vi "Eurotherm_PID.vi"() -> ()   [LabVIEW 2013]
uses:
  <vilib>/Utility/file.llb/Write To Spreadsheet File (string).vi
  <vilib>/Utility/file.llb/Write To Spreadsheet File (DBL).vi
panel:
  in  "Thermocouple\nType":u8(ring)=1 items=["J.tc", "K.tc", "L.tc", "R.tc", "B.tc", "N.tc", "T.tc", "S.tc", "PL2.tc", "C.tc", "RTD", "Lin.mV", "Lin.V", "Lin.mA", "Sr.V", "Sr.mA", "mV.C", "V.C", "mA.C"]
  in  "Ramp-Down Rate(°C/ min)":dbl
  in  "Target Setpoint (°C)":sgl format="%#.1f"
  in  "RAMP":bool
  in  "Dwell Time (min)":dbl
  in  "Ramp-Up Rate (°C/ min)":dbl
  in  "SET":bool
  in  "DELAY":u32=300 caption="ms"
  in  "Save Button":bool
  in  "File Path":path
  in  "Sample":string
  in  "User":string
  out "Time":dbl caption="(s)"
  in  "Setpoint Value":sgl min=0 max=1300 format="%.3f"
  in  "SET":bool
  in  "P":sgl=1.0
  in  "I":u32=10000
  in  "D":u32=1000
  in  "Controller Mode":u8(ring) items=["Auto", "Manual"]
  in  "stop":bool
  out "Temperature":cluster{dbl[], sgl[]}(graph)
  out "Temperature":sgl caption="°C" format="%.3g"
  in  "Unit":u8=1
  in  "VISA resource name":refnum<visa-resource-name>="COM4"
  # "Configuration - Requires Restart"
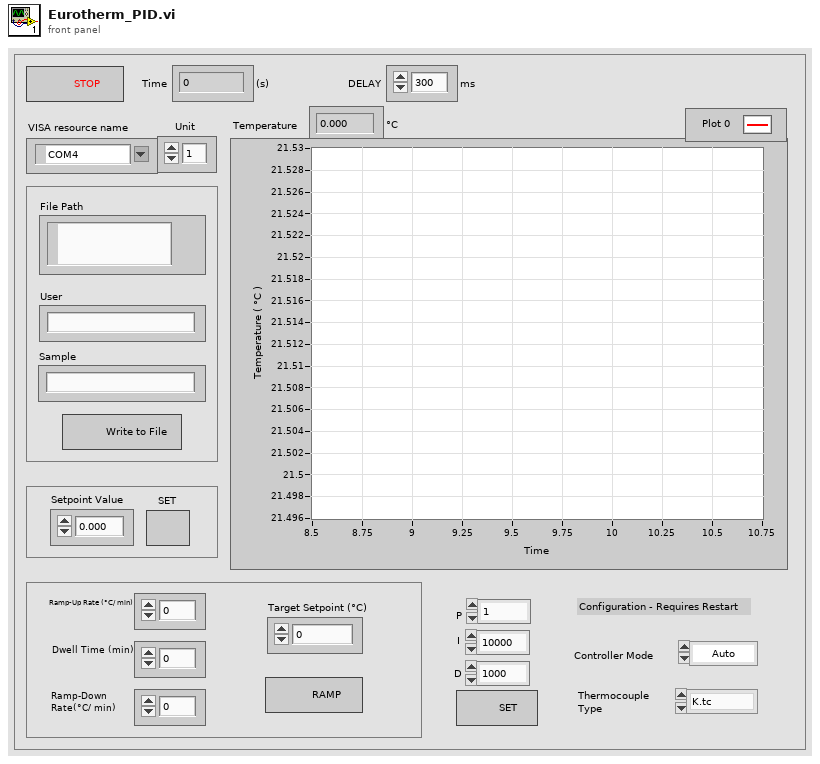
[diagram p1: front panel]
types:
  T1 = cluster{"Baud Rate (9600)":u32, "Parity (0: None)":u16, "Break Length (0)":u16}
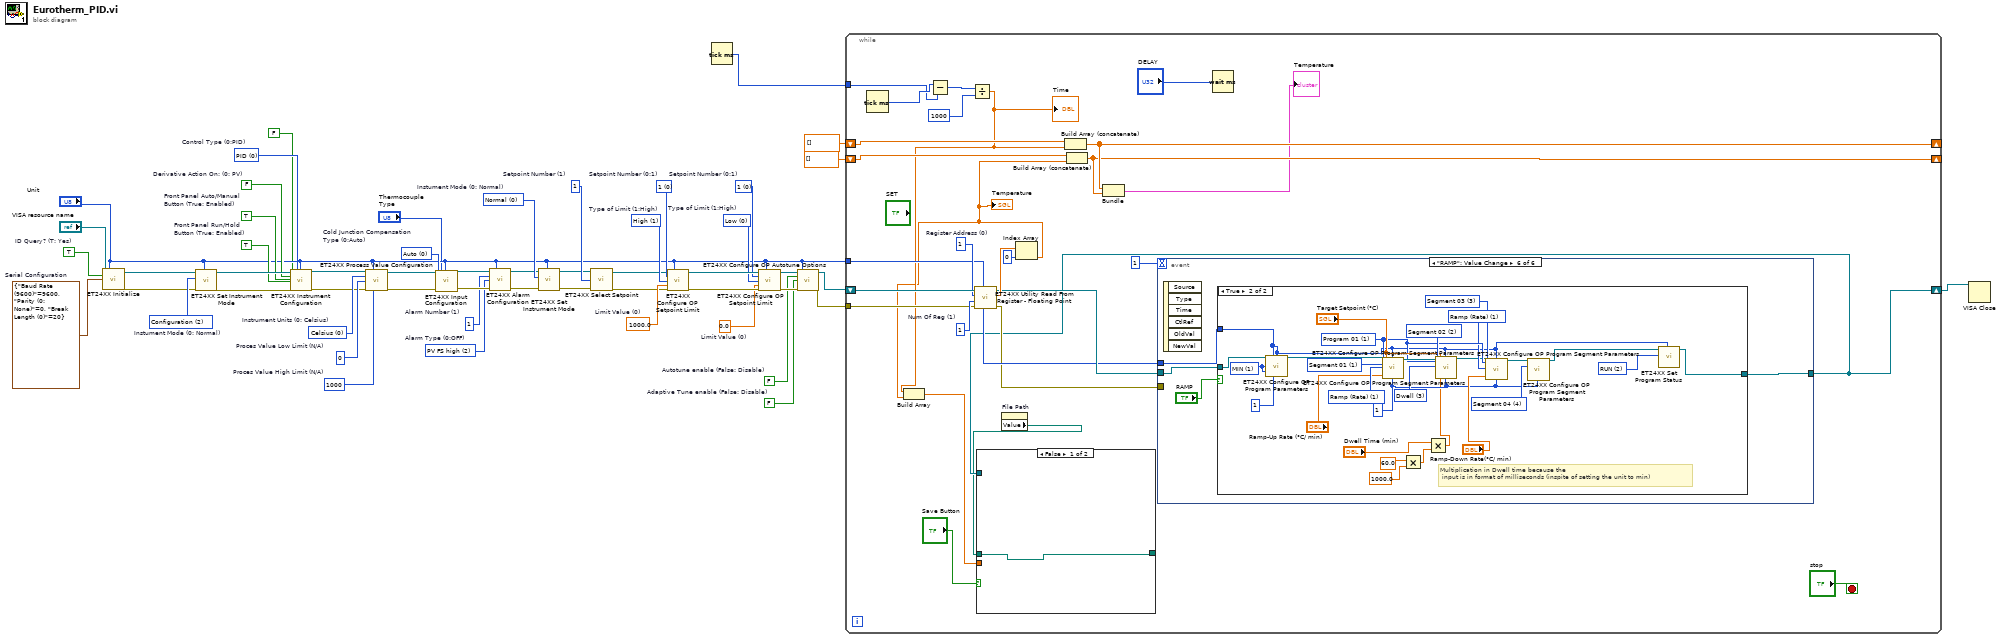
[diagram p0: block diagram]
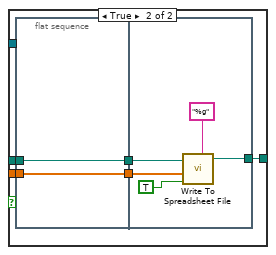
[diagram p2: hidden frame]
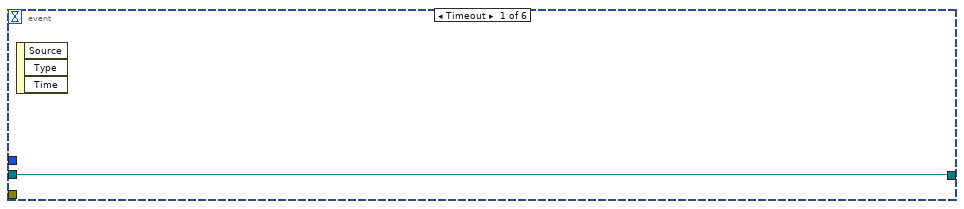
[diagram p3: hidden frame]
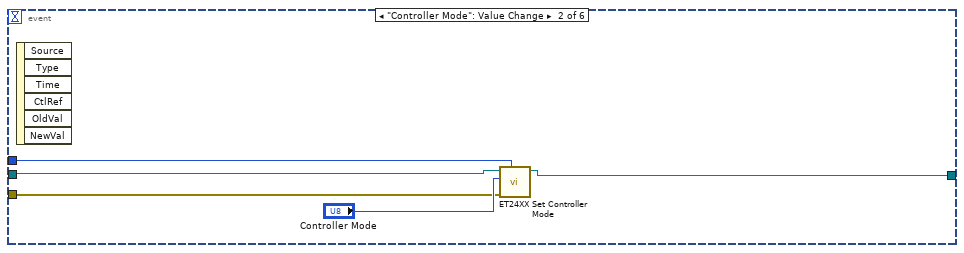
[diagram p4: hidden frame]
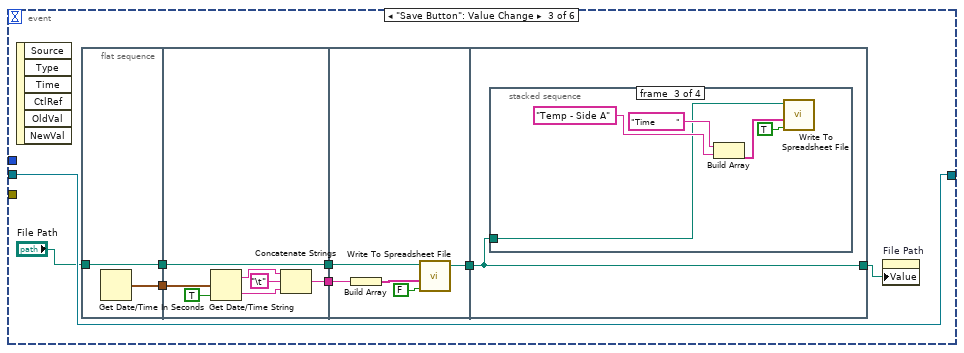
[diagram p5: hidden frame]
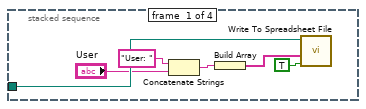
[diagram p6: hidden frame]
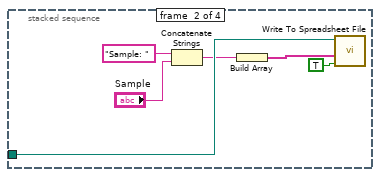
[diagram p7: hidden frame]
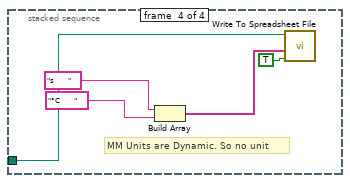
[diagram p8: hidden frame]
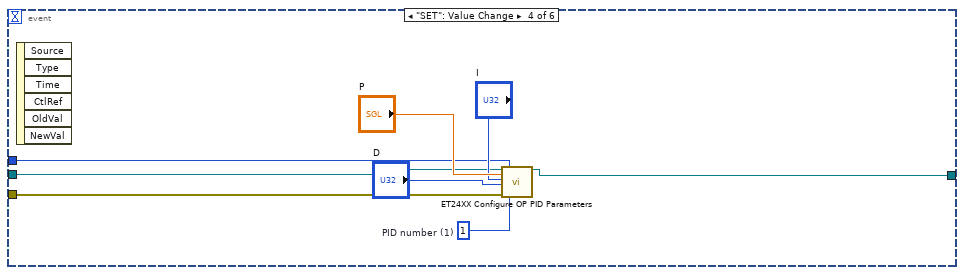
[diagram p9: hidden frame]
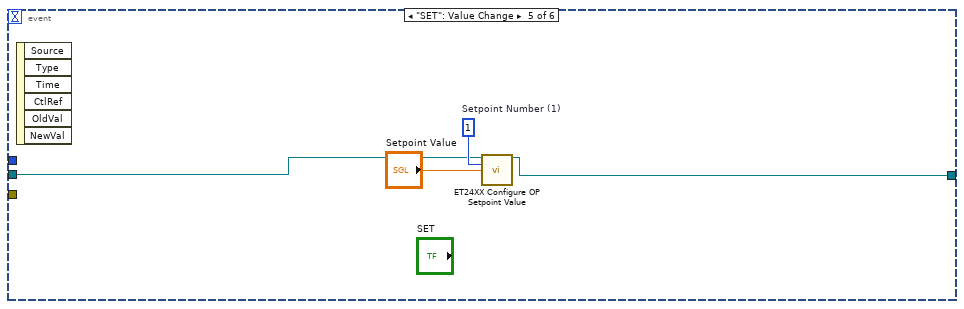
[diagram p10: hidden frame]
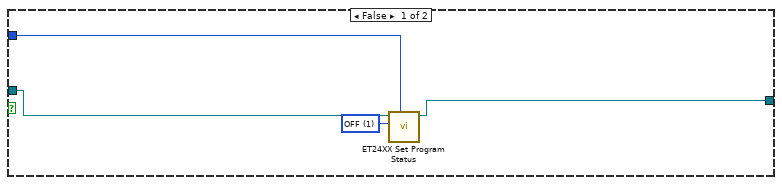
[diagram p11: hidden frame]
diagram:
  w16 = sgl 0.0  # Limit Value (0)
  w17 = i16 0 items=["Low", "High"]  # Type of Limit (1:High)
  w18 = i16 0 items=["1", "2 to 16"]  # Setpoint Number (0:1)
  w19 = sgl 1000.0  # Limit Value (0)
  w20 = i16 1 items=["Low", "High"]  # Type of Limit (1:High)
  w21 = i16 0 items=["1", "2 to 16"]  # Setpoint Number (0:1)
  w22 = i16 1  # Setpoint Number (1)
  w28 = T1 {"Baud Rate (9600)"=9600, "Parity (0: None)"=0, "Break Length (0)"=20}  # Serial Configuration
  w30 = TRUE  # ID Query? (T: Yes)
  w12 = FALSE  # Adaptive Tune enable (False: Disable)
  w13 = FALSE  # Autotune enable (False: Disable)
  w31 = TRUE  # Front Panel Auto/Manual Button (True: Enabled)
  w32 = TRUE  # Front Panel Run/Hold Button (True: Enabled)
  w33 = FALSE  # Derivative Action On: (0: PV)
  w42 = u8 2 items=["OFF"=0, "PV FS low"=1, "PV FS high"=2, "PV Dev. band"=16, "PV Dev. high"=17, "PV Dev. low"=18, "Load Current low"=34, "Load Current high"=35, "I2 FS low"=36, "I2 FS high"=37, "Wo. out. low"=38, "Wo. out. high"=39, "Wo. SP low"=40, "Wo. SP high"=41, "Rate of change"=64]  # Alarm Type (0:OFF)
  w43 = u8 1  # Alarm Number (1)
  w46 = u8 0 items=["PID", "ON/OFF", "Manual", "VP", "VP b"]  # Control Type (0:PID)
  w47 = u8 0 items=["Auto", "0 Celsius degree", "45 Celsius degree", "50 Celsius degree", "OFF"]  # Cold Junction Compensation Type (0:Auto)
  w49 = i16 1000  # Proces Value High Limit (N/A)
  w50 = i16 0  # Proces Value Low Limit (N/A)
  w51 = u8 0 items=["Celsius", "Fahrenheit", "Kelvin", "None"]  # Instrument Units (0: Celsius)
  w52 = u8 0 items=["Normal", "StandBy", "Configuration"]  # Instument Mode (0: Normal)
  w53 = u8 2 items=["Normal", "StandBy", "Configuration"]  # Instument Mode (0: Normal)
  n1 = call <userlib>:"ET24XX Initialize.vi"("VISA resource name"="VISA resource name", "Unit Address (1)"="Unit", "ID Query? (T: Yes)"=w30, "Serial Configuration"=w28) -> ("VISA resource name out"=w37:refnum<visa-resource-name>, "error out"=w38:errorcluster)  [unwired: 10 in]
  n2 = call <userlib>:"ET24XX Set Instrument Mode.vi"("Unit Address (1)"="Unit", "error in (no error)"=w38, "Instrument Mode (0: Normal)"=w53, "VISA resource name"=w37) -> ("error out"=w39:errorcluster, "VISA resource name out"=w36:refnum<visa-resource-name>)  [unwired: 6 in]
  n3 = call <userlib>:"ET24XX Instrument Configuration.vi"("VISA resource name"=w36, "Derivative Action On: (False: PV)"=w33, "Front Panel Auto/Manual\nButton (True: Enabled)"=w31, "Front Panel Run/Hold\nButton (True: Enabled)"=w32, "error in (no error)"=w39, "Control Action (True: Direct)"=FALSE, "Control Type (0: PID)"=w46, "Unit Address (1)"="Unit") -> ("VISA resource name out"=w41:refnum<visa-resource-name>, "error out"=w40:errorcluster)  [unwired: 18 in]
  n4 = call <userlib>:"ET24XX Process Value Configuration.vi"("VISA resource name"=w41, "Unit Address (1)"="Unit", "Instrument Units (0: Celsius)"=w51, "Process Value Low Limit (0)"=w50, "error in (no error)"=w40, "Process Value High Limit (0)"=w49) -> ("VISA resource name out"=w2:refnum<visa-resource-name>, "error out"=w48:errorcluster)  [unwired: 8 in]
  n5 = call <userlib>:"ET24XX Input Configuration.vi"("VISA resource name"=w2, "Cold Junction Compensation\nType (0:Auto)"=w47, "error in (no error)"=w48, "Input Type (0:J.tc)"="Thermocouple\nType", "Unit Address (1)"="Unit") -> ("VISA resource name out"=w45:refnum<visa-resource-name>, "error out"=w44:errorcluster)  [unwired: 13 in]
  n6 = call <userlib>:"ET24XX Alarm Configuration.vi"("VISA resource name"=w45, "Unit Address (1)"="Unit", "Alarm Number (1)"=w43, "Alarm Type (0:OFF)"=w42, "error in (no error)"=w44) -> ("VISA resource name out"=w35:refnum<visa-resource-name>, "error out"=w34:errorcluster)  [unwired: 9 in]
  n7 = call <userlib>:"ET24XX Set Instrument Mode.vi"("Unit Address (1)"="Unit", "error in (no error)"=w34, "Instrument Mode (0: Normal)"=w52, "VISA resource name"=w35) -> ("error out"=w27:errorcluster, "VISA resource name out"=w3:refnum<visa-resource-name>)  [unwired: 6 in]
  n8 = call <userlib>:"ET24XX Select Setpoint.vi"("VISA resource name"=w3, "Setpoint Number (1)"=w22, "error in (no error)"=w27) -> ("VISA resource name out"=w15:refnum<visa-resource-name>, "error out"=w14:errorcluster)  [unwired: 11 in]
  n9 = call <userlib>:"ET24XX Configure OP Setpoint Limit.vi"("VISA resource name"=w15, "Unit Address (1)"="Unit", "Setpoint Number (0:1)"=w21, "Type of Limit (1:High)"=w20, "Limit Value (0)"=w19, "error in (no error)"=w14) -> ("VISA resource name out"=w23:refnum<visa-resource-name>, "error out"=w26:errorcluster)  [unwired: 8 in]
  n10 = Tick Count (ms)() -> (millisecond timer value=w8:u32)
  n11 = call <userlib>:"ET24XX Configure OP Setpoint Limit.vi"("VISA resource name"=w23, "Unit Address (1)"="Unit", "Setpoint Number (0:1)"=w18, "Type of Limit (1:High)"=w17, "Limit Value (0)"=w16, "error in (no error)"=w26) -> ("VISA resource name out"=w24:refnum<visa-resource-name>, "error out"=w25:errorcluster)  [unwired: 8 in]
  n12 = call <userlib>:"ET24XX Configure OP Autotune Options.vi"("VISA resource name"=w24, "Unit Address (1)"="Unit", "Autotune enable (False: Disable)"=w13, "Adaptive Tune enable (False: Disable)"=w12, "error in (no error)"=w25) -> ("VISA resource name out"=w11:refnum<visa-resource-name>, "error out"=w6:errorcluster)  [unwired: 9 in]
  n13 = while {
    tunnel: "Unit" -> [w66]
    shift-right: [w70] -> _
    shift-left: sgl[] [] -> [w75]
    tunnel: w8 -> [w57]
    shift-right: [w71] -> _
    shift-left: dbl[] [] -> [w72]
    shift-right: [w55] -> w1
    shift-left: w11 -> [w80]
    tunnel: w6 -> [w65]
    stop <- "stop" stop-if-true
    w78 = u16 1  # Num Of Reg (1)
    w79 = u16 1  # Register Address (0)
    n14 = Tick Count (ms)() -> (millisecond timer value=w58:u32)
    n15 = Subtract(x=w58, y=w57) -> (x-y=w74:u32)
    n16 = Divide(x=w74, y=u32 1000) -> (x/y=w62:dbl)
    "Time" <- w62
    n17 = call <userlib>:"ET24XX Utility Read From Register - Floating Point.vi"("Unit Address (1)"=w66, "error in (no error)"=w65, "Num Of Reg (1)"=w78, "Register Address (0)"=w79, "VISA session"=w80) -> ("error out"=w64:errorcluster, "Data"=w77:sgl[], "dup VISA session"=w67:refnum<visa-resource-name>)  [unwired: 4 in]
    n18 = property on="File Path" class="Path"() -> ("Value"=w54:path)  [unwired: 2 in, 2 out]
    n19 = Index Array(array=w77, index=0) -> (element=w61:sgl)
    "Temperature" <- w61
    n20 = Build Array(w62, w61) -> (w60:dbl[])
    n21 = Build Array (concatenate)(w72, w62) -> (w71:dbl[])
    n22 = Build Array (concatenate)(w75, w61) -> (w70:sgl[])
    n23 = Bundle(w71, w70) -> (→"Temperature":cluster{dbl[], sgl[]})  [unwired: 1 in]
    n24 = event shown="[5] \"RAMP\": Value Change" {
      selector: _ -> [_ _ _ _ _ _]
      dyn-events: _ -> [_ _ _ _ _ _]
      timeout: 1 -> [_ _ _ _ _ _]
      tunnel: w67 -> [w94 w99 w102 w148 w155 w160]
      tunnel: [w94 w97 w102 w147 w154 w158] -> w55
      tunnel: w66 -> [_ w96 _ w146 _ w159]
      tunnel: w64 -> [_ w95 _ w145 _ _]
      event Timeout {
        n25 = event-data() -> ()  [unwired: 1 in, 3 out]
      }
      event "Controller Mode": Value Change {
        n26 = event-data() -> ()  [unwired: 1 in, 6 out]
        n27 = call <userlib>:"ET24XX Set Controller Mode.vi"("Unit Address (1)"=w96, "error in (no error)"=w95, "Controller Mode (0: Auto)"="Controller Mode", "VISA resource name"=w99) -> ("VISA resource name out"=w97:refnum<visa-resource-name>)  [unwired: 6 in, 1 out]
      }
      event "Save Button": Value Change {
        n28 = event-data() -> ()  [unwired: 1 in, 6 out]
        n29 = flat-sequence {
          tunnel: [w108] -> w107
          tunnel: [w109] -> w106
          tunnel: "File Path" -> [w109]
          tunnel: w107 -> [w114]
          tunnel: [w113] -> w105
          tunnel: [w110] -> w104
          tunnel: w106 -> [w110]
          tunnel: w105 -> [w120]
          tunnel: w104 -> [w118]
          tunnel: [w117] -> w103
          tunnel: [w122] -> w100
          tunnel: w103 -> [w122]
          frame #0 {
            n30 = Get Date/Time In Seconds() -> (seconds since 1Jan1904=w108:timestamp)
          }
          frame #1 {
            n31 = Get Date/Time String(seconds (now)=w114, want seconds? (F)=TRUE) -> (date string=w116:string, time string=w112:string)  [unwired: 1 in]
            n32 = Concatenate Strings(w116, "\t", w112) -> (w113:string)
          }
          frame #2 {
            n33 = Build Array(w120) -> (w119:string[])
            n34 = call-poly <vilib>:"Write To Spreadsheet File.vi"("append to file? (new file:F)"=FALSE ("transpose? (no:F)"), "1D data"=w119, "file path (dialog if empty)"=w118) -> ("new file path (Not A Path if cancelled)"=w117:path)  [unwired: 5 in]
          }
          frame #3 {
            n35 = stacked-sequence {
              tunnel: w122 -> [w126 w132 w135 w142]
              frame #0 {
                n36 = Concatenate Strings("User: ", "User") -> (w125:string)
                n37 = Build Array(w125) -> (w127:string[])
                n38 = call-poly <vilib>:"Write To Spreadsheet File.vi"("append to file? (new file:F)"=TRUE ("transpose? (no:F)"), "1D data"=w127, "file path (dialog if empty)"=w126) -> ()  [unwired: 5 in, 1 out]
              }
              frame #1 {
                n39 = Concatenate Strings("Sample: ", "Sample") -> (w131:string)
                n40 = Build Array(w131) -> (w133:string[])
                n41 = call-poly <vilib>:"Write To Spreadsheet File.vi"("append to file? (new file:F)"=TRUE ("transpose? (no:F)"), "1D data"=w133, "file path (dialog if empty)"=w132) -> ()  [unwired: 5 in, 1 out]
              }
              frame #2 {
                n42 = Build Array("Time       ", "Temp - Side A") -> (w138:string[])
                n43 = call-poly <vilib>:"Write To Spreadsheet File.vi"("append to file? (new file:F)"=TRUE ("transpose? (no:F)"), "1D data"=w138, "file path (dialog if empty)"=w135) -> ()  [unwired: 5 in, 1 out]
              }
              frame #3 {
                # "MM Units are Dynamic. So no unit"
                n44 = Build Array("s       ", "°C       ") -> (w143:string[])
                n45 = call-poly <vilib>:"Write To Spreadsheet File.vi"("append to file? (new file:F)"=TRUE ("transpose? (no:F)"), "1D data"=w143, "file path (dialog if empty)"=w142) -> ()  [unwired: 5 in, 1 out]
              }
            }
          }
        }
        n46 = property on="File Path" class="Path"("Value"=w100) -> ()  [unwired: 2 in, 2 out]
      }
      event "SET": Value Change {
        w152 = i16 1  # PID number (1)
        n47 = event-data() -> ()  [unwired: 1 in, 6 out]
        n48 = call <userlib>:"ET24XX Configure OP PID Parameters.vi"("VISA resource name"=w148, "Proportional Band (1)"="P", "Integral Time (ms) (0)"="I", "Derivative Time (ms) (0)"="D", "error in (no error)"=w145, "Unit Address (1)"=w146, "PID number (1)"=w152) -> ("VISA resource name out"=w147:refnum<visa-resource-name>)  [unwired: 11 in, 1 out]
      }
      event "SET": Value Change {
        w156 = i16 1  # Setpoint Number (1)
        n49 = event-data() -> ()  [unwired: 1 in, 6 out]
        n50 = call <userlib>:"ET24XX Configure OP Setpoint Value.vi"("VISA resource name"=w155, "Setpoint Number (1)"=w156, "Setpoint Value (0)"="Setpoint Value") -> ("VISA resource name out"=w154:refnum<visa-resource-name>)  [unwired: 11 in, 1 out]
      }
      event "RAMP": Value Change {
        n51 = event-data() -> ()  [unwired: 1 in, 6 out]
        n52 = case shown="True" "RAMP" {
          tunnel: w160 -> [w164 w190]
          tunnel: w159 -> [w163 w178]
          tunnel: [w161 w191] -> w158
          frame False {
            w162 = u8 1 items=["OFF"=1, "RUN"=2, "HOLD"=4] ("Program Status (1: OFF)")
            n53 = call <userlib>:"ET24XX Set Program Status.vi"("Unit Address (1)"=w163, "Program Status (1: OFF)"=w162, "VISA resource name"=w164) -> ("VISA resource name out"=w161:refnum<visa-resource-name>)  [unwired: 7 in, 1 out]
          }
          frame True {
            w173 = u16 4 items=["Segment 01"=1, "Segment 02"=2, "Segment 03"=3, "Segment 04"=4, "Segment 05"=5, "Segment 06"=6, "Segment 07"=7, "Segment 08"=8, "Segment 09"=9, "Segment 10"=10, "Segment 11"=11, "Segment 12"=12, "Segment 13"=13, "Segment 14"=14, "Segment 15"=15, "Segment 16"=16] ("Selected Segment Number \n(1: Segment1)")
            w170 = u16 1 ("Sub-Program Cycles (0)")
            w179 = u16 3 items=["Segment 01"=1, "Segment 02"=2, "Segment 03"=3, "Segment 04"=4, "Segment 05"=5, "Segment 06"=6, "Segment 07"=7, "Segment 08"=8, "Segment 09"=9, "Segment 10"=10, "Segment 11"=11, "Segment 12"=12, "Segment 13"=13, "Segment 14"=14, "Segment 15"=15, "Segment 16"=16] ("Selected Segment Number \n(1: Segment1)")
            w180 = u8 1 items=["End", "Ramp (Rate)", "Ramp (Time to Target)", "Dwell", "Step", "Call"] ("Segment Type (0: End)")
            w183 = u8 3 items=["End", "Ramp (Rate)", "Ramp (Time to Target)", "Dwell", "Step", "Call"] ("Segment Type (0: End)")
            w184 = u16 2 items=["Segment 01"=1, "Segment 02"=2, "Segment 03"=3, "Segment 04"=4, "Segment 05"=5, "Segment 06"=6, "Segment 07"=7, "Segment 08"=8, "Segment 09"=9, "Segment 10"=10, "Segment 11"=11, "Segment 12"=12, "Segment 13"=13, "Segment 14"=14, "Segment 15"=15, "Segment 16"=16] ("Selected Segment Number \n(1: Segment1)")
            w186 = u8 1 items=["End", "Ramp (Rate)", "Ramp (Time to Target)", "Dwell", "Step", "Call"] ("Segment Type (0: End)")
            w181 = u16 1 items=["Program 01"=1, "Program 02"=2, "Program 03"=3, "Program 04"=4, "Program 05"=5, "Program 06"=6, "Program 07"=7, "Program 08"=8, "Program 09"=9, "Program 10"=10, "Program 11"=11, "Program 12"=12, "Program 13"=13, "Program 14"=14, "Program 15"=15, "Program 16"=16, "Program 17"=17, "Program 18"=18, "Program 19"=19, "Program 20"=20] ("Selected Program Number \n(1: Program 01)")
            w187 = u16 1 items=["Segment 01"=1, "Segment 02"=2, "Segment 03"=3, "Segment 04"=4, "Segment 05"=5, "Segment 06"=6, "Segment 07"=7, "Segment 08"=8, "Segment 09"=9, "Segment 10"=10, "Segment 11"=11, "Segment 12"=12, "Segment 13"=13, "Segment 14"=14, "Segment 15"=15, "Segment 16"=16] ("Selected Segment Number \n(1: Segment1)")
            w189 = u8 1 items=["SEC", "MIN", "HOUR"] ("Ramp Time Units (0: SEC)")
            w192 = u8 2 items=["OFF"=1, "RUN"=2, "HOLD"=4] ("Program Status (1: OFF)")
            # "Multiplication in Dwell time because the\n input is in format of milliseconds (inspite of setting the unit to min)"
            n54 = call <userlib>:"ET24XX Configure OP Program Parameters.vi"("VISA resource name"=w190, "Unit Address (1)"=w178, "Program number (1)"=w178, "Ramp Time Units (0: SEC)"=w189, "Dwell Time Units (0: SEC)"=w189, "Program Cycles (0)"=u16 1) -> ("VISA resource name out"=w188:refnum<visa-resource-name>)  [unwired: 8 in, 1 out]
            n55 = call "ET24XX Configure OP Program Segment Parameters.vi"("VISA resource name"=w188, "Selected Program Number \n(1: Program 01)"=w181, "Selected Segment Number \n(1: Segment1)"=w187, "Segment Type (0: End)"=w186, "Ramp Rate (1)"="Ramp-Up Rate (°C/ min)", "Target Setpoint (0)"="Target Setpoint (°C)", "Unit Address (1)"=w178, "Sub-Program Cycles (0)"=w170) -> ("VISA resource name out"=w185:refnum<visa-resource-name>)  [unwired: 18 in, 1 out]
            n56 = Multiply(x=60.0, y=1000.0) -> (x*y=w166:dbl)
            n57 = Multiply(x="Dwell Time (min)", y=w166) -> (x*y=w165:dbl)
            n58 = call "ET24XX Configure OP Program Segment Parameters.vi"("VISA resource name"=w185, "Selected Program Number \n(1: Program 01)"=w181, "Selected Segment Number \n(1: Segment1)"=w184, "Segment Type (0: End)"=w183, "Target Setpoint (0)"="Target Setpoint (°C)", "Duration (N/A)"=w165, "Unit Address (1)"=w178, "Sub-Program Cycles (0)"=w170) -> ("VISA resource name out"=w177:refnum<visa-resource-name>)  [unwired: 18 in, 1 out]
            n59 = call "ET24XX Configure OP Program Segment Parameters.vi"("VISA resource name"=w177, "Selected Program Number \n(1: Program 01)"=w181, "Selected Segment Number \n(1: Segment1)"=w179, "Segment Type (0: End)"=w180, "Ramp Rate (1)"="Ramp-Down Rate(°C/ min)", "Unit Address (1)"=w178, "Sub-Program Cycles (0)"=w170) -> ("VISA resource name out"=w175:refnum<visa-resource-name>)  [unwired: 19 in, 1 out]
            n60 = call "ET24XX Configure OP Program Segment Parameters.vi"("VISA resource name"=w175, "Selected Segment Number \n(1: Segment1)"=w173, "Sub-Program Cycles (0)"=w170) -> ("VISA resource name out"=w174:refnum<visa-resource-name>)  [unwired: 23 in, 1 out]
            n61 = call <userlib>:"ET24XX Set Program Status.vi"("Unit Address (1)"=w178, "Program Status (1: OFF)"=w192, "VISA resource name"=w174) -> ("VISA resource name out"=w191:refnum<visa-resource-name>)  [unwired: 7 in, 1 out]
          }
        }
      }
    }
    n62 = case shown="False" "Save Button" {
      tunnel: [w81 w86] -> _
      tunnel: w54 -> [w81 w84]
      tunnel: w60 -> [_ w82]
      tunnel: w55 -> [_ _]
      frame False {
      }
      frame True {
        n63 = flat-sequence {
          tunnel: [w88] -> w85
          tunnel: w84 -> [w88]
          tunnel: [w87] -> w83
          tunnel: w82 -> [w87]
          tunnel: [w92] -> w86
          tunnel: w85 -> [w91]
          tunnel: w83 -> [w90]
          frame #0 {
          }
          frame #1 {
            n64 = call-poly <vilib>:"Write To Spreadsheet File.vi"("format (%.3f)"="%g", "append to file? (new file:F)"=TRUE ("transpose? (no:F)"), "1D data"=w90, "file path (dialog if empty)"=w91) -> ("new file path (Not A Path if cancelled)"=w92:path)  [unwired: 4 in]
          }
        }
      }
    }
    n65 = Wait (ms)(milliseconds to wait="DELAY") -> ()  [unwired: 1 out]
  }
  n66 = VISA Close(VISA resource name=w1) -> ()  [unwired: 1 in, 1 out]
